vi "TestApply.vi"() -> ()   [LabVIEW 2021]
uses:
  <vilib>/Instr/_visa.llb/VISA Configure Serial Port (Instr).vi
panel:
  out "Booléen":bool
  in  "VISA resource name":refnum<visa-resource-name> caption="PORT DSCUSB"
  in  "stop":bool
  out "buffer de lecture":string
  in  "Chaîne déroulante":string(combo)
  in  "VALIDER APPLY A":bool
  in  "VALIDER APPLY B":bool
  in  "Poids A":dbl
  in  "Poids B":dbl
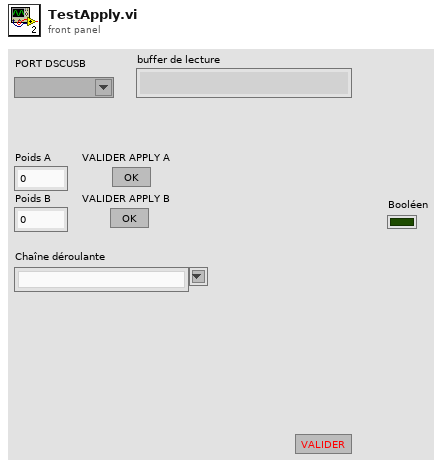
[diagram p1: front panel]
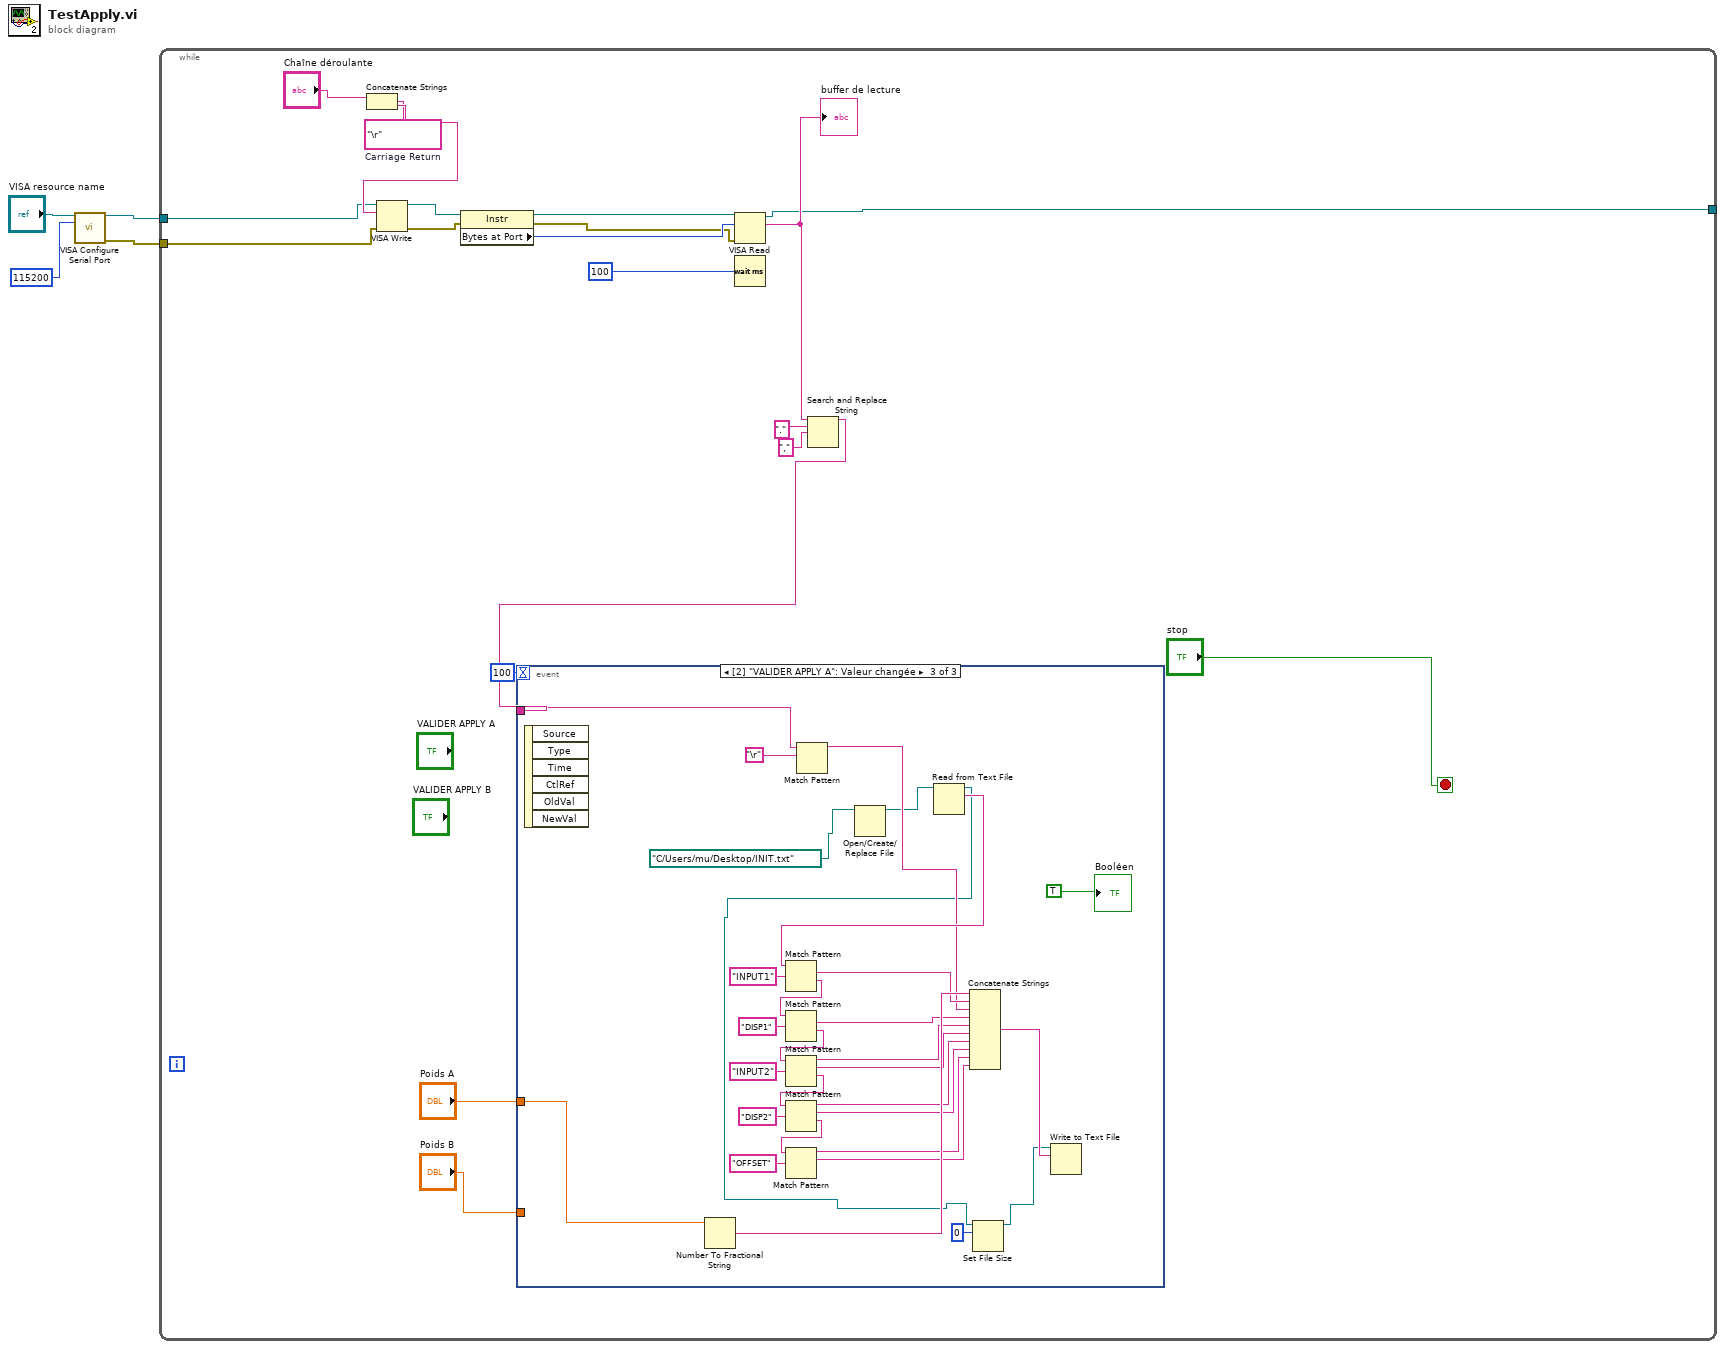
[diagram p0: block diagram]
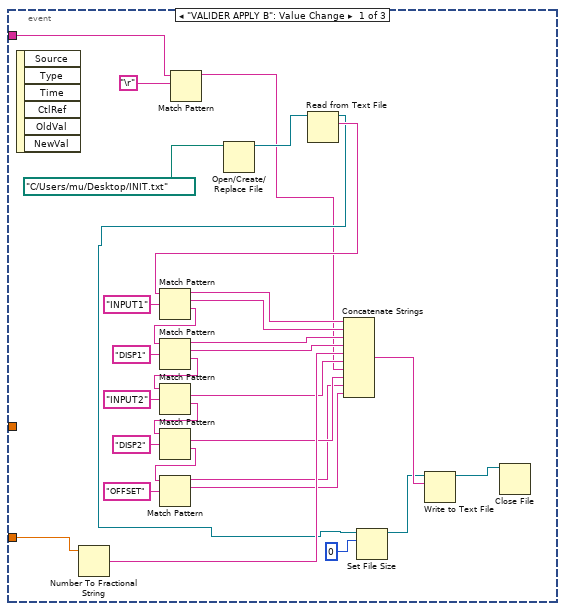
[diagram p2: hidden frame]
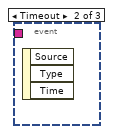
[diagram p3: hidden frame]
diagram:
  n1 = call-poly "VISA Configure Serial Port"("VISA resource name"="VISA resource name", "baud rate (9600)"=u32 115200) -> ("VISA resource name out"=w2:refnum<visa-resource-name>, "error out"=w1:errorcluster)  [unwired: 12 in]
  n2 = while {
    tunnel: [w12] -> _
    tunnel: w2 -> [w11]
    tunnel: w1 -> [w10]
    stop <- "stop" stop-if-true
    w19 = "\r"  # Carriage Return
    n3 = Concatenate Strings("Chaîne déroulante", w19) -> (w18:string)
    n4 = VISA Write(VISA resource name=w11, write buffer=w18, error in (no error)=w10) -> (VISA resource name out=w24:refnum<visa-resource-name>, error out=w23:errorcluster)  [unwired: 1 out]
    n5 = property class="Instr"(reference=w24, error in=w23) -> (reference out=w22:refnum<visa-resource-name>, error out=w20:errorcluster, "Bytes at Port"=w21:u32)
    n6 = VISA Read(VISA resource name=w22, byte count=w21, error in (no error)=w20) -> (VISA resource name out=w12:refnum<visa-resource-name>, read buffer=w14:string)  [unwired: 2 out]
    "buffer de lecture" <- w14
    n7 = Wait (ms)(milliseconds to wait=u32 100 ("attente (ms)")) -> ()  [unwired: 1 out]
    n8 = Search and Replace String(input string=w14, search string=".", replace string=",") -> (result string=w7:string)  [unwired: 5 in, 3 out]
    n9 = event shown="[2] \"VALIDER APPLY A\": Valeur changée" {
      selector: _ -> [_ _ _]
      dyn-events: _ -> [_ _ _]
      timeout: 100 -> [_ _ _]
      tunnel: w7 -> [w27 _ w72]
      tunnel: "Poids B" -> [w38 _ _]
      tunnel: "Poids A" -> [_ _ w71]
      event "VALIDER APPLY B": Value Change {
        n10 = event-data() -> ()  [unwired: 1 in, 6 out]
        n11 = Number To Fractional String(number=w38) -> (F-format string=w37:string)  [unwired: 3 in]
        n12 = Match Pattern(string=w27, regular expression="\r") -> (before substring=w25:string)  [unwired: 1 in, 3 out]
        n13 = Open/Create/Replace File(file path (use dialog)=path "C:/Users/mu/Desktop/INIT.txt" ("chemin du fichier (utiliser une boîte de dialogue)")) -> (refnum out=w53:refnum<file>)  [unwired: 5 in, 2 out]
        n14 = Read from Text File(file (use dialog)=w53) -> (refnum out=w29:refnum<file>, text=w43:string)  [unwired: 3 in, 2 out]
        n15 = Match Pattern(string=w43, regular expression="INPUT1" ("expression régulière")) -> (before substring=w42:string, match substring=w41:string, after substring=w51:string)  [unwired: 1 in, 1 out]
        n16 = Match Pattern(string=w51, regular expression="DISP1" ("expression régulière")) -> (before substring=w40:string, match substring=w39:string, after substring=w48:string)  [unwired: 1 in, 1 out]
        n17 = Match Pattern(string=w48, regular expression="INPUT2" ("expression régulière")) -> (match substring=w36:string, after substring=w47:string)  [unwired: 1 in, 2 out]
        n18 = Match Pattern(string=w47, regular expression="DISP2" ("expression régulière")) -> (match substring=w35:string, after substring=w44:string)  [unwired: 1 in, 2 out]
        n19 = Match Pattern(string=w44, regular expression="OFFSET" ("expression régulière")) -> (before substring=w34:string, match substring=w33:string)  [unwired: 1 in, 2 out]
        n20 = Concatenate Strings(w42, w41, w40, w39, w37, w36, w25, w35, w34, w33) -> (w32:string)
        n21 = Set File Size(6:i64 0 ("taille (en octets)"), 7:w29) -> (3:w28:refnum<file>)  [unwired: 1 in, 1 out]
        n22 = Write to Text File(file (use dialog)=w28, text=w32) -> (refnum out=w31:refnum<file>)  [unwired: 2 in, 2 out]
        n23 = Close File(refnum=w31) -> ()  [unwired: 1 in, 2 out]
      }
      event Timeout {
        n24 = event-data() -> ()  [unwired: 1 in, 3 out]
      }
      event "VALIDER APPLY A": Value Change {
        n25 = event-data() -> ()  [unwired: 1 in, 6 out]
        n26 = Number To Fractional String(number=w71) -> (F-format string=w70:string)  [unwired: 3 in]
        n27 = Match Pattern(string=w72, regular expression="\r") -> (before substring=w68:string)  [unwired: 1 in, 3 out]
        n28 = Open/Create/Replace File(file path (use dialog)=path "C:/Users/mu/Desktop/INIT.txt" ("chemin du fichier (utiliser une boîte de dialogue)")) -> (refnum out=w56:refnum<file>)  [unwired: 5 in, 2 out]
        n29 = Read from Text File(file (use dialog)=w56) -> (refnum out=w60:refnum<file>, text=w83:string)  [unwired: 3 in, 2 out]
        n30 = Match Pattern(string=w83, regular expression="INPUT1" ("expression régulière")) -> (match substring=w69:string, after substring=w79:string)  [unwired: 1 in, 2 out]
        n31 = Match Pattern(string=w79, regular expression="DISP1" ("expression régulière")) -> (match substring=w67:string, after substring=w80:string)  [unwired: 1 in, 2 out]
        n32 = Match Pattern(string=w80, regular expression="INPUT2" ("expression régulière")) -> (before substring=w66:string, match substring=w65:string, after substring=w81:string)  [unwired: 1 in, 1 out]
        n33 = Match Pattern(string=w81, regular expression="DISP2" ("expression régulière")) -> (before substring=w64:string, match substring=w63:string, after substring=w82:string)  [unwired: 1 in, 1 out]
        n34 = Match Pattern(string=w82, regular expression="OFFSET" ("expression régulière")) -> (before substring=w62:string, match substring=w61:string)  [unwired: 1 in, 2 out]
        n35 = Concatenate Strings(w70, w69, w68, w67, w66, w65, w64, w63, w62, w61) -> (w84:string)
        n36 = Set File Size(6:i64 0 ("taille (en octets)"), 7:w60) -> (3:w59:refnum<file>)  [unwired: 1 in, 1 out]
        n37 = Write to Text File(file (use dialog)=w59, text=w84) -> ()  [unwired: 2 in, 3 out]
        "Booléen" <- TRUE
      }
    }
  }
